vi "Write reference.vi"(8 "error in (no error)":errorcluster, 10 "new reference":refnum<k24>, 11 "MelsecTCP in":refnum<class "MelsecFxLinks.lvclass">) -> (0 "error out":errorcluster, 3 "MelsecTCP out":refnum<class "MelsecFxLinks.lvclass">)   [LabVIEW 2020, in "MelsecFxLinks.lvclass"]
uses:
  MelsecFxLinks.lvclass
  C:/Users/Fred Guo/Desktop/API_Salcomp_CMES/Libraries/HslCommunication/HslCommunication.dll
  HslCommunication.dll
  MelsecFxLinks.lvclass/MelsecFxLinks.ctl
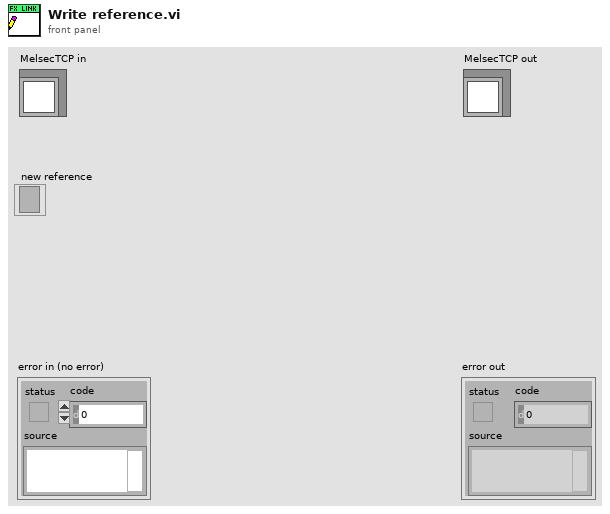
[diagram p1: front panel]
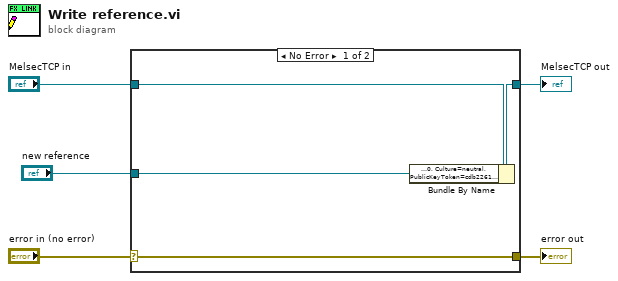
[diagram p0: block diagram]
diagram:
  n1 = case shown="No Error" "error in (no error)" {
    selector: "error in (no error)" -> [w9 w10]
    tunnel: [w9 w10] -> w4
    tunnel: [w7 w11] -> w2
    tunnel: "MelsecTCP in" -> [w8 w11]
    tunnel: "new reference" -> [w6 _]
    frame No Error {
      n2 = Bundle By Name(cluster=w8, "new reference"=w6) -> (w7:refnum<class "MelsecFxLinks.lvclass">)
    }
    frame Error {
    }
  }
  "error out" <- w4
  "MelsecTCP out" <- w2
